vi "getCost.vi"(8 "error in (no error)":errorcluster, 11 "Soy in":refnum<class "Soy.lvclass">) -> (0 "error out":errorcluster, 2 "cost":dbl, 3 "Soy out":refnum<class "Soy.lvclass">)   [LabVIEW 2016, in "Soy.lvclass"]
uses:
  Soy.lvclass
  CondimentDecorator/CondimentDecorator.lvclass
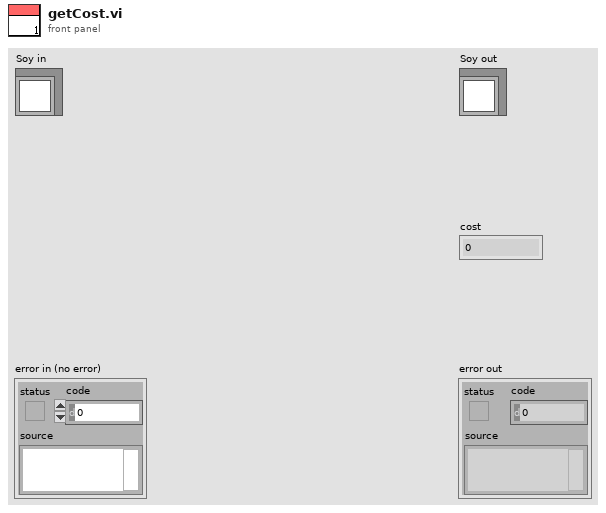
[diagram p1: front panel]
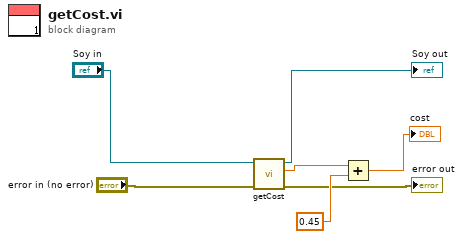
[diagram p0: block diagram]
diagram:
  n1 = call-parent "getCost.vi"("error in (no error)"="error in (no error)", "CondimentDecorator in"="Soy in") -> ("error out"=→"error out":errorcluster, "cost"=w1:dbl, "CondimentDecorator out"=→"Soy out":refnum<class "Soy.lvclass">)  [unwired: 7 in]
  n2 = Add(x=w1, y=0.45 ("cost")) -> (x+y=→"cost":dbl)
